vi "Get Session Property.vi"   [LabVIEW 2020, in "SLSC.lvlib"]
uses:
  <vilib>/SLSC/SLSC.lvlib
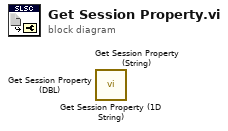
[diagram p0: block diagram]
diagram:
  n1 = call <vilib>:"Get Session Property (1D String).vi"() -> ()  [unwired: 13 in, 3 out]
  n2 = call <vilib>:"Get Session Property (String).vi"() -> ()  [unwired: 13 in, 3 out]
  n3 = call <vilib>:"Get Session Property (DBL).vi"() -> ()  [unwired: 13 in, 3 out]
